vi "Remote Client Metrics.vi"() -> ()   [LabVIEW 2016]
panel:
  in  "stop":bool
  out "time":cluster{i32[], i32[]}[](graph)
  in  "Number of Messages":i32=20
  in  "step":dbl
  in  "end":dbl
  in  "start":dbl
  out "throughput":cluster{i32[], dbl[]}[](graph)
  out "message rate":cluster{i32[], dbl[]}[](graph)
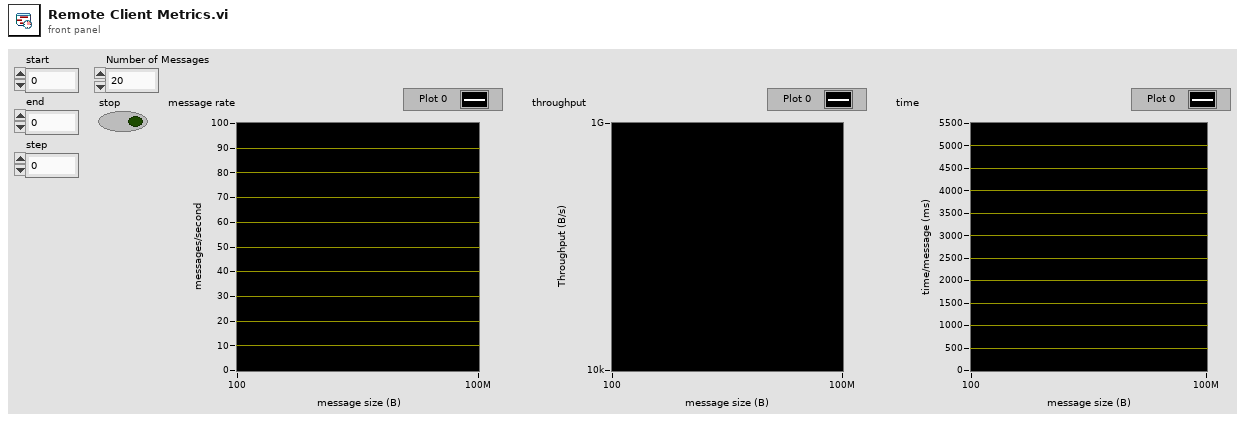
[diagram p1: front panel]
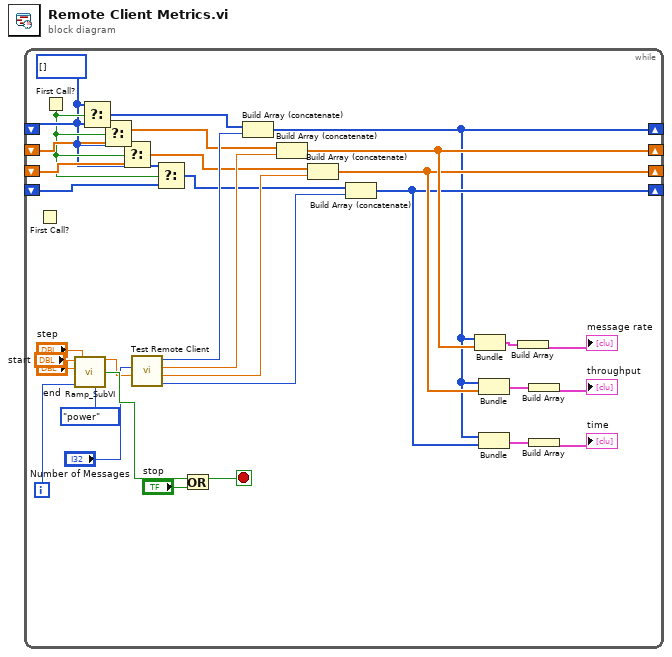
[diagram p0: block diagram]
diagram:
  n1 = while {
    shift-right: [w10] -> _
    shift-left: _ -> [w24]
    shift-right: [w16] -> _
    shift-left: _ -> [w22]
    shift-right: [w15] -> _
    shift-left: _ -> [w23]
    shift-right: [w14] -> _
    shift-left: _ -> [w11]
    i -> [w32]
    stop <- w2 stop-if-true
    w3 = i32[] [] ("t")
    n2 = First Call?() -> ()  [unwired: 1 out]
    n3 = First Call?() -> (First Call?: T/F=w17:bool)
    n4 = call <userlib>:"Ramp_SubVI.vi"("Enum"=enum16{"linear", "power"}."power", "index"=w32, "step"="step", "end"="end", "start"="start") -> ("Stop?"=w33:bool, "Numeric"=w13:dbl)
    n5 = Select(t=w3, s=w17, f=w24) -> (s? t:f=w21:i32[])
    n6 = Select(t=w3, s=w17, f=w22) -> (s? t:f=w20:dbl[])
    n7 = Select(t=w3, s=w17, f=w23) -> (s? t:f=w19:dbl[])
    n8 = call "Test Remote Client.vi"("Array size"=w13, "Number of Messages"="Number of Messages") -> ("<time/message (ms)>"=w25:i32, "bytes/second"=w26:dbl, "messages/second"=w27:dbl, "<size>"=w28:i32)  [unwired: 6 in]
    n9 = Select(t=w3, s=w17, f=w11) -> (s? t:f=w18:i32[])
    n10 = Or(x=w33, y="stop") -> (x .or. y?=w2:bool)
    n11 = Build Array (concatenate)(w21, w28) -> (w10:i32[])
    n12 = Build Array (concatenate)(w20, w27) -> (w16:dbl[])
    n13 = Build Array (concatenate)(w19, w26) -> (w15:dbl[])
    n14 = Build Array (concatenate)(w18, w25) -> (w14:i32[])
    n15 = Bundle(w10, w16) -> (w9:cluster{i32[], dbl[]})  [unwired: 1 in]
    n16 = Bundle(w10, w15) -> (w7:cluster{i32[], dbl[]})  [unwired: 1 in]
    n17 = Bundle(w10, w14) -> (w6:cluster{i32[], i32[]})  [unwired: 1 in]
    n18 = Build Array(w9) -> (→"message rate":cluster{i32[], dbl[]}[])
    n19 = Build Array(w7) -> (→"throughput":cluster{i32[], dbl[]}[])
    n20 = Build Array(w6) -> (→"time":cluster{i32[], i32[]}[])
  }
